vi "output.vi"(8 "error in":errorcluster, 10 "data table in":T1, 11 "Modbus Slave runtime in":refnum<class "Modbus Module runtime.lvclass">) -> (0 "error out":errorcluster, 2 "data table out":T1, 3 "Modbus Slave runtime out":refnum<class "Modbus Module runtime.lvclass">)   [LabVIEW 2013, in "Modbus Module runtime.lvclass"]
doc: "Provides an interface for writing data to a module at runtime. While this interface performs no operations, a child should provide an override which may write to any open sessions, references, or interfaces.Platypus Framework 1.0.1.65\nNI Systems Engineering - National Instruments"
uses:
  Modbus Module runtime.lvclass
  <vilib>/NI/Tag Bus/table/data table.ctl
  Modbus Module runtime.lvclass/Modbus Module runtime.ctl
  <vilib>/NI/Modbus Library/API/Modbus API.lvclass
  <vilib>/NI/Modbus Library/API/Slave/Modbus Slave.lvclass
  <vilib>/NI/Tag Bus/table/data table.lvlib
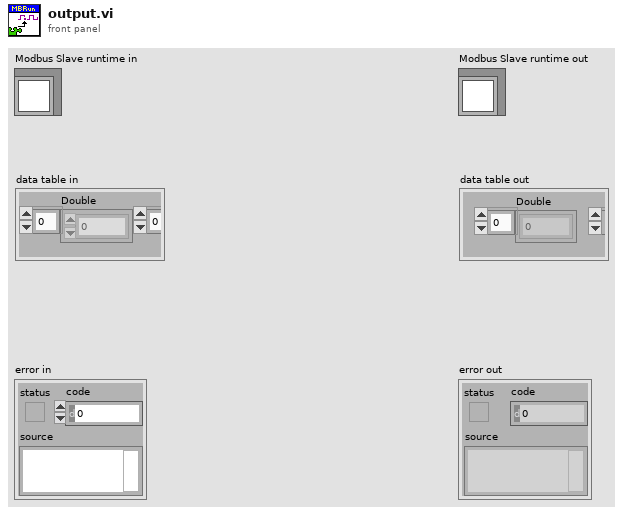
[diagram p1: front panel]
types:
  T1 = typedef "tag bus.lvlib/data table.lvlib/data table.ctl" = cluster{"Double":dbl[], "Single":sgl[], "I64":i64[], "I32":i32[], "I16":i16[], "I8":i8[], "U64":u64[], "U32":u32[], "U16":u16[], "U8":u8[], "Boolean":bool[], "String":string[], "Array of Double":cluster{"DBL Array":dbl[]}[], "Array of Single":cluster{"SGL Array":sgl[]}[], "Array of I64":cluster{"I64 Array":i64[]}[], "Array of I32":cluster{"I32 Array":i32[]}[], "Array of I16":cluster{"I16 Array":i16[]}[], "Array of I8":cluster{"I8 Array":i8[]}[], "Array of U64":cluster{"U64 Array":u64[]}[], "Array of U32":cluster{"U32 Array":u32[]}[], "Array of U16":cluster{"U16 Array":u16[]}[], "Array of U8":cluster{"U8 Array":u8[]}[], "Array of Boolean":cluster{"Boolean Array":bool[]}[], "Array of String":cluster{"String Array":string[]}[]}
  T2 = typedef "Modbus Slave runtime.lvclass/output bulk data access.ctl" = cluster{"modbus type":T3, "start":u16, "length":u16, "maps":T4[], "coils":bool[], "registers":u16[]}
  T3 = typedef "Modbus Module Channel.lvclass/data bank type.ctl" = enum16{"coils", "discrete inputs", "input registers", "holding registers"}
  T4 = typedef "Modbus Slave runtime.lvclass/data mapping elements.ctl" = cluster{"data type":T5, "data index":i32, "element index":i32, "subindex/regcount":i32}
  T5 = typedef "tag bus.lvlib/tag descriptor.lvclass/Data Type.ctl" = enum16{"Double", "Single", "I64", "I32", "I16", "I8", "U64", "U32", "U16", "U8", "Boolean", "String", "Array of Double", "Array of Single", "Array of I64", "Array of I32", "Array of I16", "Array of I8", "Array of U64", "Array of U32", "Array of U16", "Array of U8", "Array of Boolean", "Array of String"}
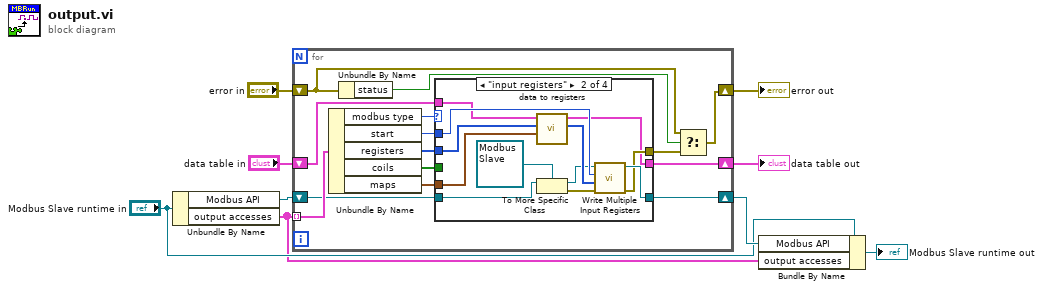
[diagram p0: block diagram]
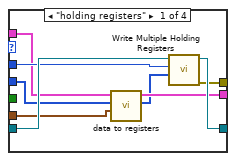
[diagram p2: hidden frame]
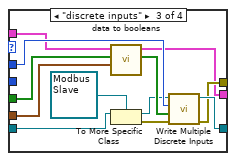
[diagram p3: hidden frame]
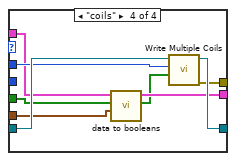
[diagram p4: hidden frame]
diagram:
  n1 = Unbundle By Name("Modbus Slave runtime in") -> ("Modbus API"=w9:refnum<class "Modbus API.lvclass">, "output accesses"=w1:T2[])
  n2 = for {
    shift-right: [w20] -> w8
    shift-left: w9 -> [w21]
    shift-right: [w23] -> w2
    shift-left: "error in" -> [w11]
    tunnel: w1 -> [w22] mode=indexing
    shift-right: [w13] -> w5
    shift-left: "data table in" -> [w14]
    n3 = Unbundle By Name(w22) -> ("modbus type"=w18:T3, "start"=w17:u16, "registers"=w16:u16[], "coils"=w15:bool[], "maps"=w12:T4[])
    n4 = Unbundle By Name(w11) -> ("status"=w10:bool)
    n5 = case shown="\"input registers\"" w18 {
      tunnel: w21 -> [w32 w34 w46 w65]
      tunnel: [w31 w44 w56 w64] -> w20
      tunnel: [w29 w42 w54 w62] -> w19
      tunnel: w17 -> [w30 w43 w55 w63]
      tunnel: w16 -> [w28 w41 _ _]
      tunnel: w15 -> [_ _ w52 w59]
      tunnel: w14 -> [w26 w40 w53 w61]
      tunnel: [w25 w39 w51 w58] -> w13
      tunnel: w12 -> [w27 w37 w49 w60]
      frame "holding registers" {
        n6 = call "data to registers.vi"("specifications"=w27, "allocation"=w28, "data table"=w26) -> ("registers"=w24:u16[], "allocation"=w25:T1)  [unwired: 7 in]
        n7 = call-dynamic "Write Multiple Holding Registers.vi"("registers to write"=w24, "starting address"=w30, "Modbus instance in"=w32) -> ("error out"=w29:errorcluster, "Modbus instance out"=w31:refnum<class "Modbus API.lvclass">)  [unwired: 7 in]
      }
      frame "input registers" {
        n8 = call "data to registers.vi"("specifications"=w37, "allocation"=w41, "data table"=w40) -> ("registers"=w38:u16[], "allocation"=w39:T1)  [unwired: 7 in]
        n9 = To More Specific Class(target class=refnum<class "Modbus Slave.lvclass"> refnum ("Modbus slave in"), reference=w34) -> (specific class reference=w35:refnum<class "Modbus Slave.lvclass">, error out=w33:errorcluster)  [unwired: 1 in]
        n10 = call-dynamic "Write Multiple Input Registers.vi"("error in"=w33, "input registers to write"=w38, "starting address"=w43, "Modbus slave in"=w35) -> ("error out"=w42:errorcluster, "Modbus slave out"=w44:refnum<class "Modbus Slave.lvclass">)  [unwired: 6 in]
      }
      frame "discrete inputs" {
        n11 = call "data to booleans.vi"("specifications"=w49, "allocation"=w52, "data table"=w53) -> ("registers"=w50:bool[], "allocation"=w51:T1)  [unwired: 7 in]
        n12 = To More Specific Class(target class=refnum<class "Modbus Slave.lvclass"> refnum ("Modbus slave in"), reference=w46) -> (specific class reference=w45:refnum<class "Modbus Slave.lvclass">, error out=w48:errorcluster)  [unwired: 1 in]
        n13 = call-dynamic "Write Multiple Discrete Inputs.vi"("error in"=w48, "discrete inputs to write"=w50, "starting address"=w55, "Modbus slave in"=w45) -> ("error out"=w54:errorcluster, "Modbus slave out"=w56:refnum<class "Modbus Slave.lvclass">)  [unwired: 6 in]
      }
      frame "coils" {
        n14 = call "data to booleans.vi"("specifications"=w60, "allocation"=w59, "data table"=w61) -> ("registers"=w57:bool[], "allocation"=w58:T1)  [unwired: 7 in]
        n15 = call-dynamic "Write Multiple Coils.vi"("coils to write"=w57, "starting address"=w63, "Modbus instance in"=w65) -> ("error out"=w62:errorcluster, "Modbus instance out"=w64:refnum<class "Modbus API.lvclass">)  [unwired: 7 in]
      }
    }
    n16 = Select(t=w11, s=w10, f=w19) -> (s? t:f=w23:errorcluster)
  }
  "error out" <- w2
  "data table out" <- w5
  n17 = Bundle By Name(cluster="Modbus Slave runtime in", "Modbus API"=w8, "output accesses"=w1) -> (→"Modbus Slave runtime out":refnum<class "Modbus Module runtime.lvclass">)
